vi "Get Pose.vi"   [LabVIEW 2018]
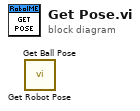
[diagram p0: block diagram]
diagram:
  n1 = call "Get Robot Pose.vi"() -> ()  [unwired: 11 in, 1 out]
  n2 = call "Get Ball Pose.vi"() -> ()  [unwired: 11 in, 1 out]
